vi "Autonomous Independent.vi"   [LabVIEW 2013]
doc: "This VI is called when autonomous begins, and will automatically be terminated when autonomous ends. You can carry out timed or sensor driven robot movement independently without needing to return to the caller."
uses:
  Robot Global Data.vi
types:
  T1 = typedef "WPI_DriverStationMatch Info.ctl" = cluster{"Autonomous Elapsed Seconds":dbl, "TeleOp Elapsed Seconds":dbl, "Disabled Elapsed Seconds":dbl, "Visited Autonomous":bool, "Visited TeleOp":bool, "Visited Disabled":bool, "Autonomous Settings":cluster{"Autonomous Style":enum16{"Iterative", "Independent"}, "VI Refnum":refnum<vi>}}
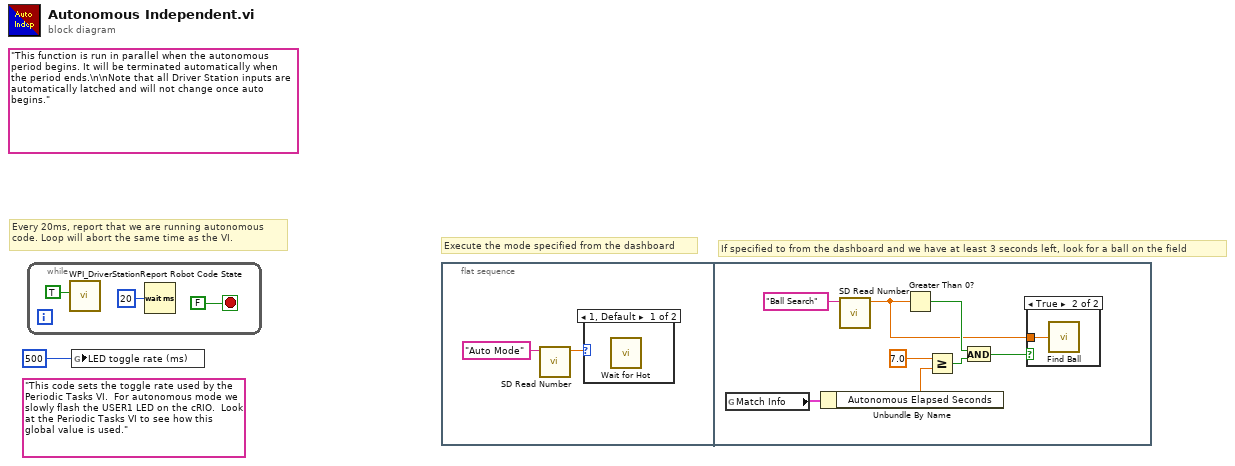
[diagram p0: block diagram]
diagram:
  (unwired) "This code sets the toggle rate used by the Periodic Tasks VI.  For autonomous mode we slowly flash the USER1 LED on the cRIO.  Look at the Periodic Tasks VI to see how this global value is used."
  (unwired) "This function is run in parallel when the autonomous period begins. It will be terminated automatically when the period ends.\n\nNote that all Driver Station inputs are automatically latched and will not change once auto begins."
  # "If specified to from the dashboard and we have at least 3 seconds left, look for a ball on the field"
  # "Execute the mode specified from the dashboard"
  # "Every 20ms, report that we are running autonomous\ncode. Loop will abort the same time as the VI."
  n1 = while {
    stop <- FALSE stop-if-true
    n2 = call <vilib>:"WPI_DriverStationReport Robot Code State.vi"("Autonomous"=TRUE) -> ()  [unwired: 10 in, 1 out]
    n3 = Wait (ms)(milliseconds to wait=u32 20) -> ()  [unwired: 1 out]
  }
  n4 = global write "Robot Global Data.vi" "LED toggle rate (ms)"(u32 500 ("LED ms toggle rate")) -> ()
  n5 = flat-sequence {
    frame #0 {
      n6 = call <vilib>:"SD Read Number.vi"("Name"="Auto Mode") -> ("Numeric"=w6:dbl)  [unwired: 8 in, 2 out]
      n7 = case shown="1, Default" w6 {
        frame 1, Default {
          n8 = call "Wait for Hot.vi"() -> ()  [unwired: 12 in]
        }
        frame 0 {
          # "Do nothing"
        }
      }
    }
    frame #1 {
      n9 = global read "Robot Global Data.vi" "Match Info"() -> (w13:T1)
      n10 = Unbundle By Name(w13) -> ("Autonomous Elapsed Seconds"=w12:dbl)
      n11 = call <vilib>:"SD Read Number.vi"("Name"="Ball Search") -> ("Numeric"=w7:dbl)  [unwired: 8 in, 2 out]
      n12 = Greater Than 0?(x=w7) -> (x > 0?=w8:bool)
      n13 = Greater Or Equal?(x=7.0, y=w12) -> (x >= y?=w10:bool)
      n14 = And(x=w8, y=w10) -> (x .and. y?=w9:bool)
      n15 = case shown="True" w9 {
        tunnel: w7 -> [_ w15]
        frame False {
        }
        frame True {
          n16 = call "Find Ball.vi"("Search Mode"=w15) -> ()
        }
      }
    }
  }
